vi "Exit.vi"(8 "error in (no error)":errorcluster, 11 "Work In":refnum<class "Work.lvclass">) -> (0 "error out":errorcluster, 3 "Work Out":refnum<class "Work.lvclass">)   [LabVIEW 2024, in "Test States.lvlib" / "Work.lvclass"]
doc: "This is an abstract method. Override this method to define the behavior when you leave the state."
uses:
  Work.lvclass
  Work.lvclass/Work.ctl
  Test State/Test State.lvclass
  <vilib>/ActorFramework/Actor/Actor.lvclass
  Test UI Messages/Update Log Msg/Update Log Msg.lvclass
  G:/Leveling/LabVIEW/Learning/Actor Framework/actor-state-machine/Test States/Test State/Test State.lvclass
  C:/Program Files/National Instruments/LabVIEW 2024/vi.lib/ni/Actors/State Actor/State Actor/State Actor.lvclass
  C:/Program Files/National Instruments/LabVIEW 2024/vi.lib/ActorFramework/Actor/Actor.lvclass
  G:/Leveling/LabVIEW/Learning/Actor Framework/actor-state-machine/Test States/Work/Work.lvclass
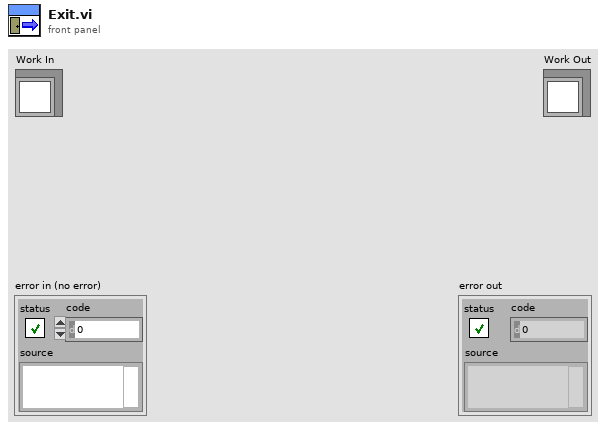
[diagram p1: front panel]
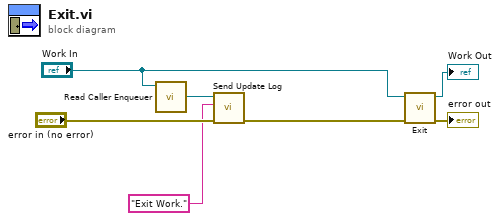
[diagram p0: block diagram]
diagram:
  n1 = call <vilib>:"Read Caller Enqueuer.vi"("Actor"="Work In") -> ("Caller Enqueuer"=w2:refnum<class "Message Enqueuer.lvclass">)  [unwired: 10 in]
  n2 = call "Send Update Log.vi"("error in (no error)"="error in (no error)", "Message"="Exit Work.", "Message Enqueuer"=w2) -> ("error out"=w3:errorcluster)  [unwired: 7 in, 1 out]
  n3 = call-parent "Exit.vi"("error in (no error)"=w3, "Old State"="Work In") -> ("error out"=→"error out":errorcluster, "New State"=→"Work Out":refnum<class "Work.lvclass">)  [unwired: 8 in]
